vi "CompareDevices.vi"(9 "New Dev array":refnum<class "Device.lvclass">[](array[class]), 10 "Old Dev array":refnum<class "Device.lvclass">[](array[class])) -> (2 "compatible?":bool)   [LabVIEW 2013]
doc: "This utility checks if two device arrays are \"compatible.\" \n\nCompatible arrays have the same number of devices, each of which matches in device class and column classes. No private data (such as table SWI, column \"functionality\", etc.) is checked.\n\nThe comparison is done linearly through the arrays by device and is stopped upon finding the first incompatibility. If a size mismatch is encountered, the internal monitors \"<array> index\" are set to -1. Otherwise, they record the index where a class mismatch occured; if no mismatch is found, index then contains the length of each matched column array."
uses:
  Device/Device.lvclass
panel:
  out "Last Col index":i32[](array[numeric])
  out "Last Dev index":i32
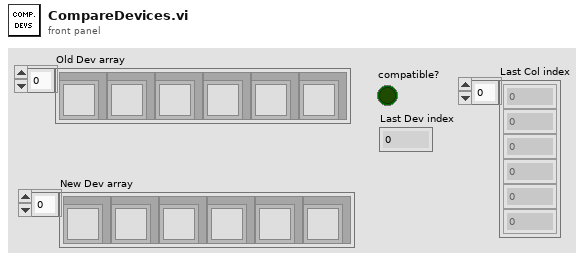
[diagram p1: front panel]
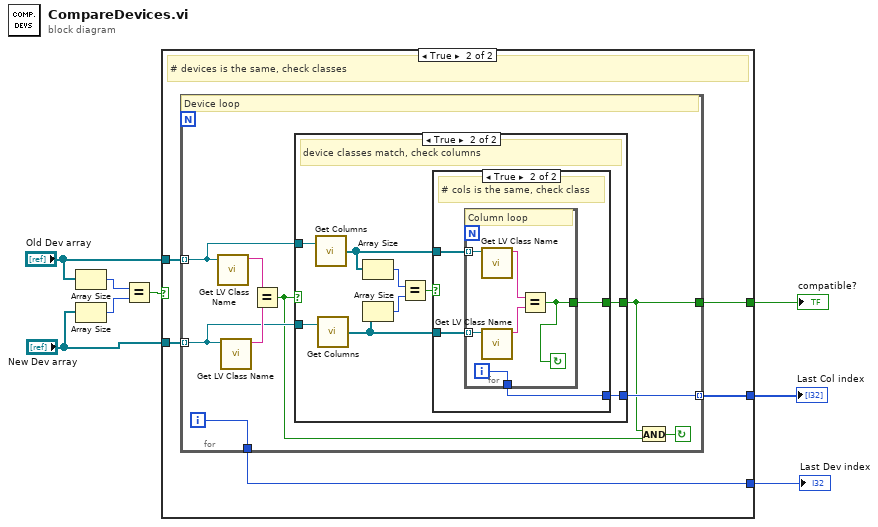
[diagram p0: block diagram]
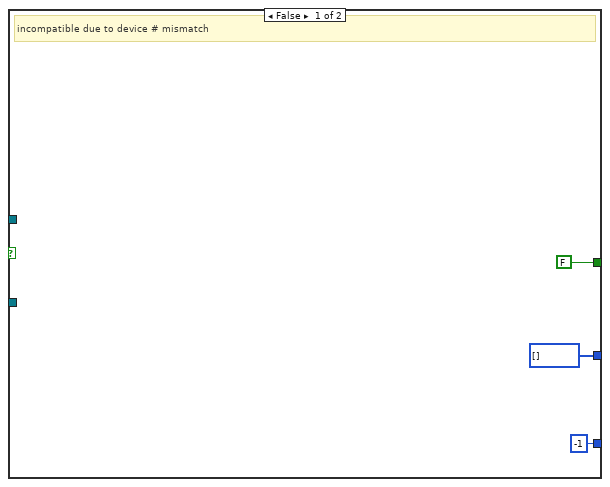
[diagram p2: hidden frame]
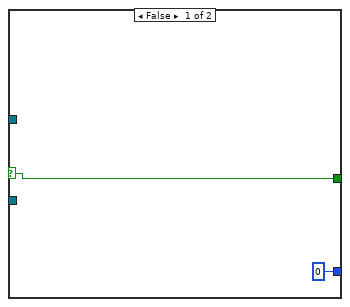
[diagram p3: hidden frame]
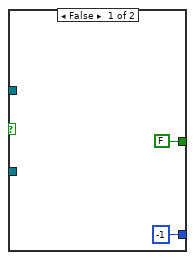
[diagram p4: hidden frame]
diagram:
  n1 = Array Size(array="Old Dev array") -> (size(s)=w7:i32)
  n2 = Array Size(array="New Dev array") -> (size(s)=w6:i32)
  n3 = Equal?(x=w7, y=w6) -> (x = y?=w5:bool)
  n4 = case shown="True" w5 {
    tunnel: [FALSE w14] -> w8
    tunnel: "Old Dev array" -> [_ w16]
    tunnel: "New Dev array" -> [_ w15]
    tunnel: [i32[] [] w13] -> w2
    tunnel: [-1 w12] -> w1
    frame False {
      # "incompatible due to device # mismatch"
    }
    frame True {
      # "# devices is the same, check classes"
      n5 = for {
        tunnel: w16 -> [w23] mode=indexing
        tunnel: w15 -> [w22] mode=indexing
        tunnel: [w18] -> w14
        tunnel: [w21] -> w12
        tunnel: [w20] -> w13 mode=indexing
        i -> [w21]
        stop <- w19 continue-if-true
        # "Device loop"
        n6 = call <vilib>:"Get LV Class Name.vi"("object"=w23) -> ("class name"=w25:string)  [unwired: 9 in, 1 out]
        n7 = call <vilib>:"Get LV Class Name.vi"("object"=w22) -> ("class name"=w24:string)  [unwired: 9 in, 1 out]
        n8 = Equal?(x=w25, y=w24) -> (x = y?=w17:bool)
        n9 = case shown="True" w17 {
          selector: w17 -> [w27 _]
          tunnel: w23 -> [_ w36]
          tunnel: w22 -> [_ w35]
          tunnel: [w27 w29] -> w18
          tunnel: [0 w28] -> w20
          frame False {
          }
          frame True {
            # "device classes match, check columns"
            n10 = call-dynamic "Get Columns.vi"("Device in"=w36) -> ("Columns"=w31:refnum<class "Column.lvclass">[])  [unwired: 1 in, 2 out]
            n11 = call-dynamic "Get Columns.vi"("Device in"=w35) -> ("Columns"=w30:refnum<class "Column.lvclass">[])  [unwired: 1 in, 2 out]
            n12 = Array Size(array=w31) -> (size(s)=w33:i32)
            n13 = Array Size(array=w30) -> (size(s)=w34:i32)
            n14 = Equal?(x=w33, y=w34) -> (x = y?=w32:bool)
            n15 = case shown="True" w32 {
              tunnel: w31 -> [_ w42]
              tunnel: w30 -> [_ w41]
              tunnel: [FALSE w40] -> w29
              tunnel: [-1 w39] -> w28
              frame False {
              }
              frame True {
                # "# cols is the same, check class"
                n16 = for {
                  tunnel: w42 -> [w48] mode=indexing
                  tunnel: w41 -> [w47] mode=indexing
                  tunnel: [w43] -> w40
                  tunnel: [w44] -> w39
                  i -> [w44]
                  stop <- w43 continue-if-true
                  # "Column loop"
                  n17 = call <vilib>:"Get LV Class Name.vi"("object"=w48) -> ("class name"=w45:string)  [unwired: 9 in, 1 out]
                  n18 = call <vilib>:"Get LV Class Name.vi"("object"=w47) -> ("class name"=w46:string)  [unwired: 9 in, 1 out]
                  n19 = Equal?(x=w45, y=w46) -> (x = y?=w43:bool)
                }
              }
            }
          }
        }
        n20 = And(x=w18, y=w17) -> (x .and. y?=w19:bool)
      }
    }
  }
  "compatible?" <- w8
  "Last Col index" <- w2
  "Last Dev index" <- w1
